vi "cm_Display State Engine.vi"(8 "error in (no error)":errorcluster, 10 "Wfm Notifier":refnum<notifier>, 11 "Message Queue":T1) -> (0 "error out":errorcluster, 1 "Message Value":string, 2 "Message Name":string, 3 "Message Queue out":T1, 4 "Data":waveform(dbl)[](array[waveform]), 5 "Exit Process":bool)   [LabVIEW 2009, in "Channel Monitor.xctl"]
uses:
  Channel Monitor.xctl
  <userlib>/AMC/subVIs/TypeDefs/amc_Message Queue.ctl
  <userlib>/AMC/subVIs/TypeDefs/amc_Message.ctl
  <userlib>/Tools/Keyed Array/Tools_KeyedArray KeyedArray.ctl
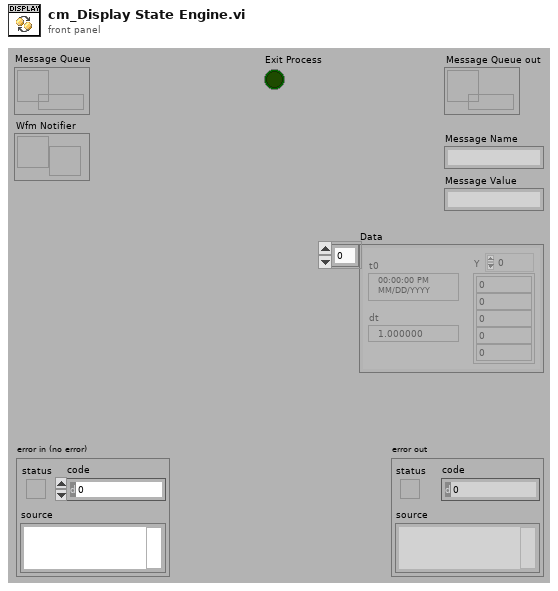
[diagram p1: front panel]
types:
  T1 = typedef "amc_Message Queue.ctl" = refnum<queue>
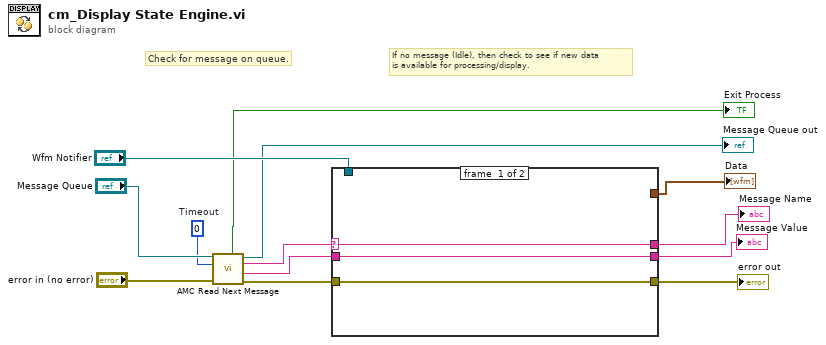
[diagram p0: block diagram]
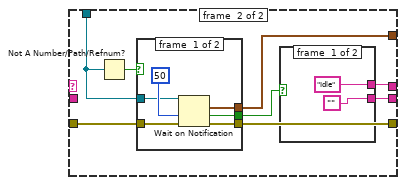
[diagram p2: hidden frame]
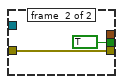
[diagram p3: hidden frame]
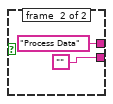
[diagram p4: hidden frame]
diagram:
  w6 = 0  # Timeout
  # "If no message (Idle), then check to see if new data\nis available for processing/display."
  # "Check for message on queue."
  n1 = call <userlib>:"AMC Read Next Message.vi"("error in (no error)"="error in (no error)", "timeout (1ms)"=w6, "Message Queue in"="Message Queue") -> ("error out"=w3:errorcluster, "Message Value"=w4:string, "Message Name"=w5:string, "Message Queue out"=→"Message Queue out":T1, "Exit Process"=→"Exit Process":bool)  [unwired: 1 in, 3 out]
  n2 = case shown="\"\", \"Idle\"" w5 {
    selector: w5 -> [w15 _]
    tunnel: w3 -> [w16 w24]
    tunnel: [w16 w23] -> w13
    tunnel: "Wfm Notifier" -> [_ w18]
    tunnel: w4 -> [w14 _]
    tunnel: [w15 w21] -> w11
    tunnel: [w14 w20] -> w10
    tunnel: [_ w19] -> w1
    frame #0 {
    }
    frame #1 {
      n3 = Not A Number/Path/Refnum?(number/path/refnum=w18) -> (NaN/Path/Refnum?=w17:bool)
      n4 = case shown="False" w17 {
        tunnel: w24 -> [w30 w32]
        tunnel: [w29 w32] -> w23
        tunnel: [w28 TRUE ("timed out?")] -> w22
        tunnel: [w26 _] -> w19
        tunnel: w18 -> [w25 _]
        frame #0 {
          n5 = Wait on Notification(notifier=w25, timeout in ms (-1)=50, error in (no error)=w30) -> (notification=w26:waveform(dbl)[], timed out?=w28:bool, error out=w29:errorcluster)  [unwired: 1 in, 1 out]
        }
        frame #1 {
        }
      }
      n6 = case shown="False" w22 {
        tunnel: ["Idle" "Process Data"] -> w21
        tunnel: ["" ""] -> w20
        frame #0 {
        }
        frame #1 {
        }
      }
    }
  }
  "error out" <- w13
  "Message Name" <- w11
  "Message Value" <- w10
  "Data" <- w1
